vi "AB_900_1000_Project_WebService_Info.vi"(6 "dataForPrevious in":T1, 7 "action":T3, 8 "error in (no error)":errorcluster, 10 "webServiceInfo in":T2, 11 "Object In":T4) -> (0 "error out":errorcluster, 2 "webServiceInfo out":T2, 3 "Object Out":T4, 4 "dataFromPrevious":T1)   [LabVIEW 2020]
uses:
  <resource>/Framework/Providers/API/ItemRef.ctl
  <vilib>/AppBuilder/RW_Project/AB_RW_Project_PropBag_Action.ctl
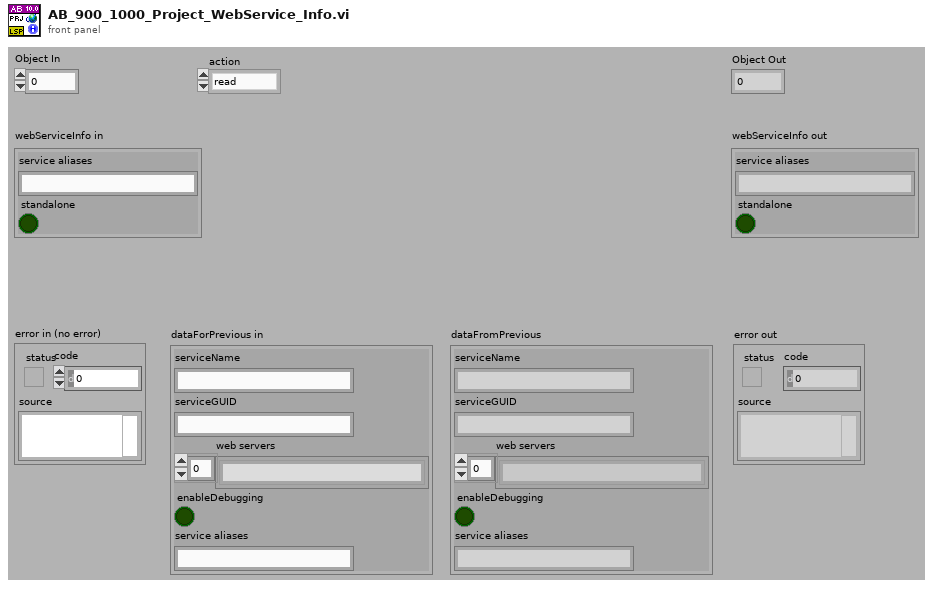
[diagram p1: front panel]
types:
  T1 = cluster{"serviceName":string, "serviceGUID":string, "web servers":string[], "enableDebugging":bool, "service aliases":string}
  T2 = cluster{"service aliases":string, "standalone":bool}
  T3 = typedef "AB_RW_Project_PropBag_Action.ctl" = enum16{"read", "write", "clear", "readPrevious", "writePrevious", "clearPrevious"}
  T4 = typedef "ItemRef.ctl" = u64
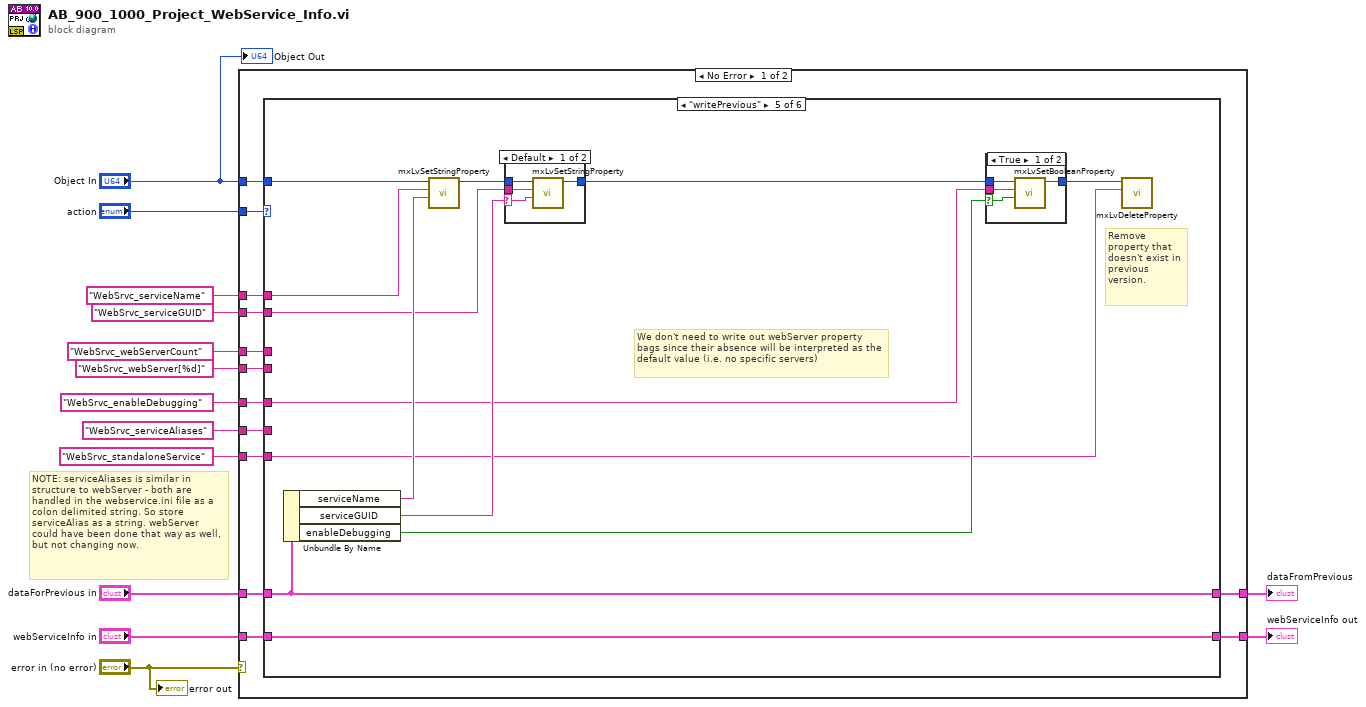
[diagram p0: block diagram]
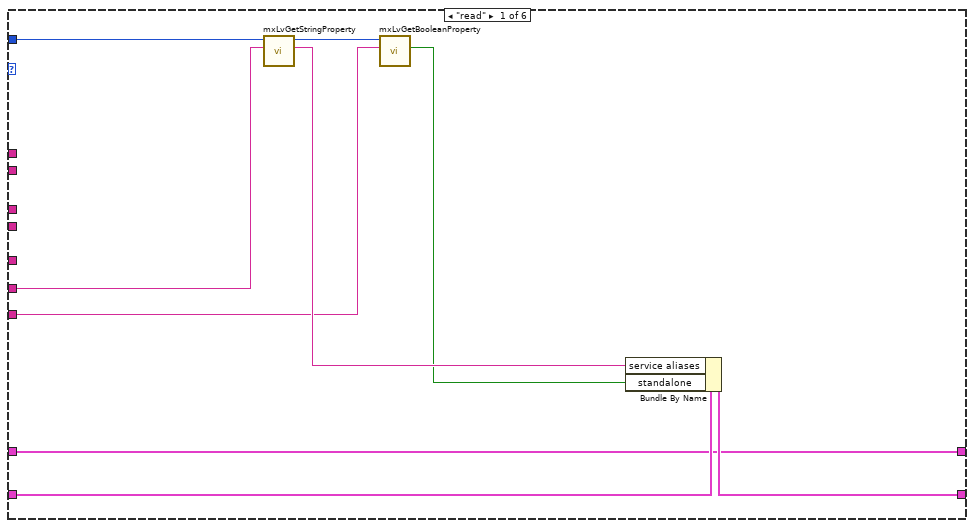
[diagram p2: hidden frame]
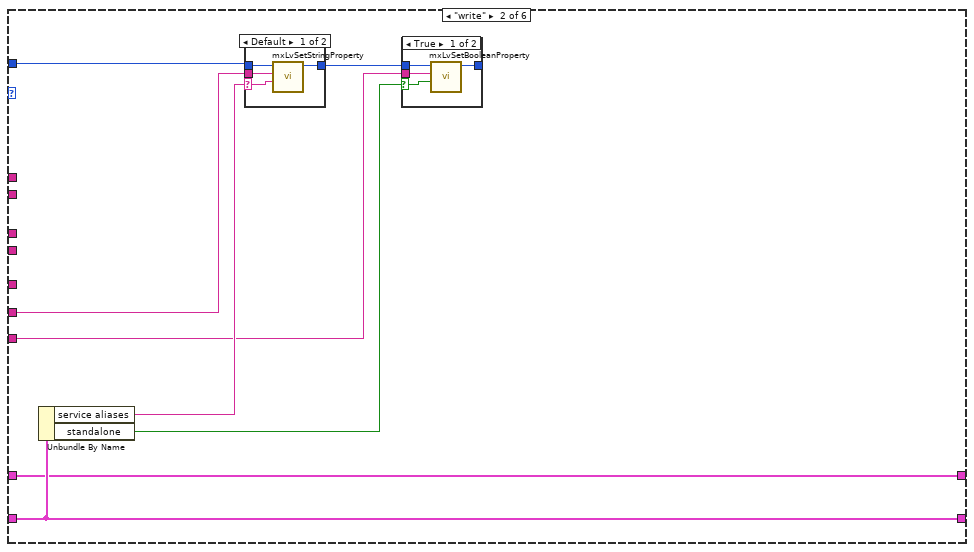
[diagram p3: hidden frame]
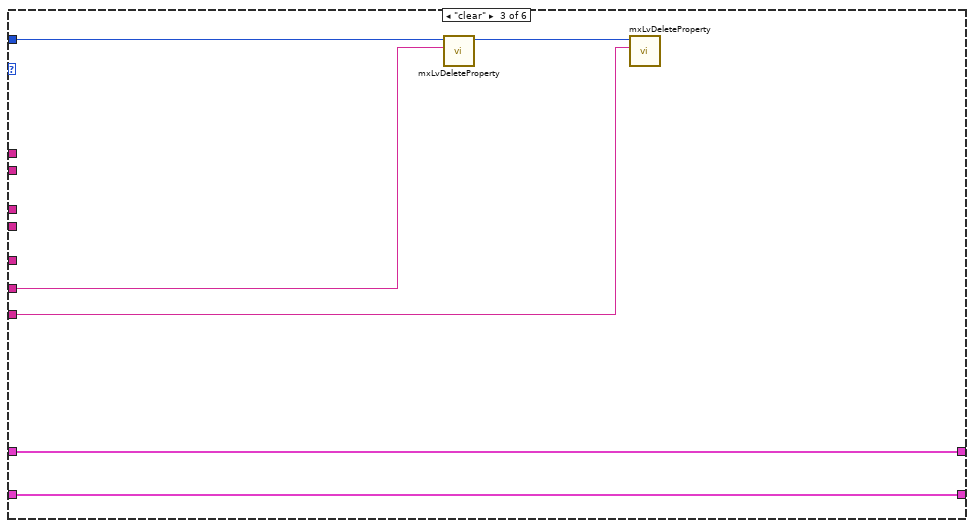
[diagram p6: hidden frame]
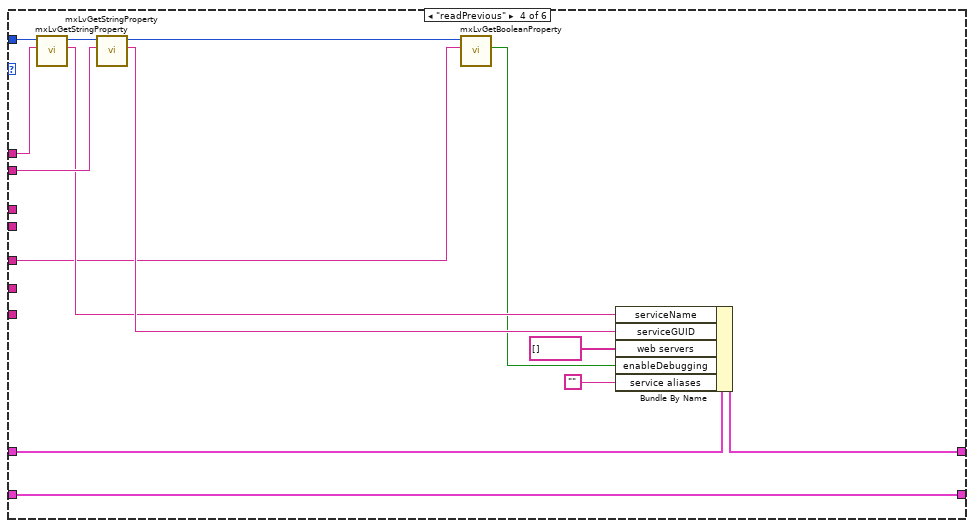
[diagram p7: hidden frame]
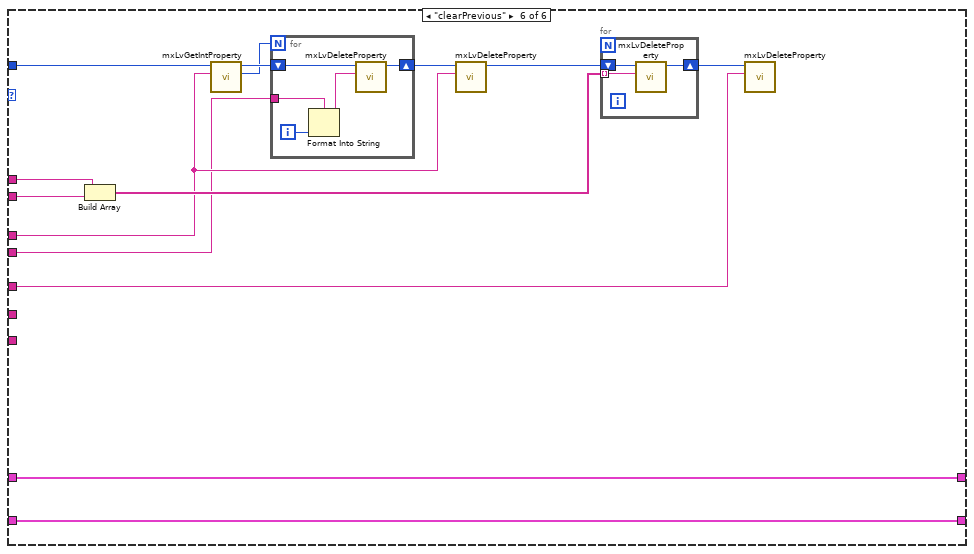
[diagram p10: hidden frame]
diagram:
  # "NOTE: serviceAliases is similar in structure to webServer - both are handled in the webservice.ini file as a colon delimited string. So store serviceAlias as a string. webServer could have been done that way as well, but not changing now."
  n1 = case shown="No Error" "error in (no error)" {
    tunnel: "Object In" -> [w27 _]
    tunnel: [w21 _] -> w6
    tunnel: "WebSrvc_serviceGUID" ("Tag") -> [w26 _]
    tunnel: "WebSrvc_webServerCount" ("Tag") -> [w25 _]
    tunnel: "WebSrvc_webServer[%d]" ("Tag") -> [w24 _]
    tunnel: "webServiceInfo in" -> [w23 _]
    tunnel: "action" -> [w22 _]
    tunnel: "WebSrvc_serviceName" ("Tag") -> [w20 _]
    tunnel: "WebSrvc_enableDebugging" ("Tag") -> [w19 _]
    tunnel: "WebSrvc_serviceAliases" ("Tag") -> [w18 _]
    tunnel: "dataForPrevious in" -> [w17 _]
    tunnel: [w16 _] -> w2
    tunnel: "WebSrvc_standaloneService" ("Tag") -> [w15 _]
    frame No Error {
      n2 = case shown="\"writePrevious\"" w22 {
        tunnel: w27 -> [w31 w43 w57 w72 w86 w101]
        tunnel: w26 -> [_ _ _ w74 w82 w111]
        tunnel: w25 -> [_ _ _ _ _ w99]
        tunnel: w24 -> [_ _ _ _ _ w98]
        tunnel: w23 -> [w35 w44 w60 w66 w87 w109]
        tunnel: [w36 w44 w60 w66 w87 w109] -> w21
        tunnel: w20 -> [_ _ _ w70 w84 w108]
        tunnel: w19 -> [_ _ _ w68 w78 w106]
        tunnel: w18 -> [w34 w42 w56 _ _ _]
        tunnel: w17 -> [w32 w41 w59 w65 w77 w105]
        tunnel: [w32 w41 w59 w64 w77 w105] -> w16
        tunnel: w15 -> [w29 w37 w55 _ w75 _]
        frame "read" {
          n3 = call <resource>:"mxLvGetStringProperty.vi"("Tag"=w34, "Item"=w31) -> ("Value"=w33:string, "Item"=w30:T4)  [unwired: 1 in, 7 out]
          n4 = call <resource>:"mxLvGetBooleanProperty.vi"("Tag"=w29, "Item"=w30) -> ("Value"=w28:bool)  [unwired: 1 in, 8 out]
          n5 = Bundle By Name(cluster=w35, "service aliases"=w33, "standalone"=w28) -> (w36:T2)
        }
        frame "write" {
          n6 = Unbundle By Name(w44) -> ("service aliases"=w40:string, "standalone"=w38:bool)
          n7 = case shown="Default" w40 {
            selector: w40 -> [w51 _]
            tunnel: w43 -> [w53 w54]
            tunnel: w42 -> [w52 _]
            tunnel: [w50 w54] -> w39
            frame Default {
              n8 = call <resource>:"mxLvSetStringProperty.vi"("Value (\"\")"=w51, "Tag"=w52, "Item"=w53) -> ("Item"=w50:T4)  [unwired: 2 in, 6 out]
            }
            frame "" {
            }
          }
          n9 = case shown="True" w38 {
            selector: w38 -> [w47 _]
            tunnel: w39 -> [w48 w49]
            tunnel: w37 -> [w46 _]
            tunnel: [w45 w49] -> _
            frame True {
              n10 = call <resource>:"mxLvSetBooleanProperty.vi"("Value (F)"=w47, "Tag"=w46, "Item"=w48) -> ("Item"=w45:T4)  [unwired: 2 in, 6 out]
            }
            frame False {
            }
          }
        }
        frame "clear" {
          n11 = call <resource>:"mxLvDeleteProperty.vi"("Tag"=w56, "Item"=w57) -> ("Item"=w58:T4)  [unwired: 1 in, 8 out]
          n12 = call <resource>:"mxLvDeleteProperty.vi"("Tag"=w55, "Item"=w58) -> ()  [unwired: 1 in, 9 out]
        }
        frame "readPrevious" {
          n13 = call <resource>:"mxLvGetStringProperty.vi"("Tag"=w70, "Item"=w72) -> ("Value"=w69:string, "Item"=w71:T4)  [unwired: 1 in, 7 out]
          n14 = call <resource>:"mxLvGetStringProperty.vi"("Tag"=w74, "Item"=w71) -> ("Value"=w73:string, "Item"=w63:T4)  [unwired: 1 in, 7 out]
          n15 = call <resource>:"mxLvGetBooleanProperty.vi"("Tag"=w68, "Item"=w63) -> ("Value"=w67:bool)  [unwired: 1 in, 8 out]
          n16 = Bundle By Name(cluster=w65, "serviceName"=w69, "serviceGUID"=w73, "web servers"=string[] [], "enableDebugging"=w67, "service aliases"="") -> (w64:T1)
        }
        frame "writePrevious" {
          # "Remove property that doesn't exist in previous version."
          # "We don't need to write out webServer property bags since their absence will be interpreted as the default value (i.e. no specific servers)"
          n17 = Unbundle By Name(w77) -> ("serviceName"=w85:string, "serviceGUID"=w81:string, "enableDebugging"=w79:bool)
          n18 = call <resource>:"mxLvSetStringProperty.vi"("Value (\"\")"=w85, "Tag"=w84, "Item"=w86) -> ("Item"=w83:T4)  [unwired: 2 in, 6 out]
          n19 = case shown="Default" w81 {
            selector: w81 -> [w93 _]
            tunnel: w83 -> [w96 w97]
            tunnel: w82 -> [w95 _]
            tunnel: [w94 w97] -> w80
            frame Default {
              n20 = call <resource>:"mxLvSetStringProperty.vi"("Value (\"\")"=w93, "Tag"=w95, "Item"=w96) -> ("Item"=w94:T4)  [unwired: 2 in, 6 out]
            }
            frame "" {
            }
          }
          n21 = case shown="True" w79 {
            selector: w79 -> [w90 _]
            tunnel: w80 -> [w91 w92]
            tunnel: w78 -> [w89 _]
            tunnel: [w88 w92] -> w76
            frame True {
              n22 = call <resource>:"mxLvSetBooleanProperty.vi"("Value (F)"=w90, "Tag"=w89, "Item"=w91) -> ("Item"=w88:T4)  [unwired: 2 in, 6 out]
            }
            frame False {
            }
          }
          n23 = call <resource>:"mxLvDeleteProperty.vi"("Tag"=w75, "Item"=w76) -> ()  [unwired: 1 in, 9 out]
        }
        frame "clearPrevious" {
          n24 = Build Array(w108, w111) -> (w110:string[])
          n25 = call <resource>:"mxLvGetIntProperty.vi"("Tag"=w99, "Item"=w101) -> ("Value"=w103:i32, "Item"=w104:T4)  [unwired: 1 in, 7 out]
          n26 = for {
            N: w103 -> [_]
            shift-right: [w113] -> w102
            shift-left: w104 -> [w114]
            tunnel: w98 -> [w115]
            i -> [w116]
            n27 = Format Into String(format string=w115, w116) -> (resulting string=w112:string)  [unwired: 2 in, 1 out]
            n28 = call <resource>:"mxLvDeleteProperty.vi"("Tag"=w112, "Item"=w114) -> ("Item"=w113:T4)  [unwired: 1 in, 8 out]
          }
          n29 = call <resource>:"mxLvDeleteProperty.vi"("Tag"=w99, "Item"=w102) -> ("Item"=w100:T4)  [unwired: 1 in, 8 out]
          n30 = for {
            tunnel: w110 -> [w118] mode=indexing
            shift-right: [w117] -> w107
            shift-left: w100 -> [w119]
            n31 = call <resource>:"mxLvDeleteProperty.vi"("Tag"=w118, "Item"=w119) -> ("Item"=w117:T4)  [unwired: 1 in, 8 out]
          }
          n32 = call <resource>:"mxLvDeleteProperty.vi"("Tag"=w106, "Item"=w107) -> ()  [unwired: 1 in, 9 out]
        }
      }
    }
    frame Error {
    }
  }
  "webServiceInfo out" <- w6
  "dataFromPrevious" <- w2
  "Object Out" <- "Object In"
  "error out" <- "error in (no error)"
